vi "setSweep.vi"(8 "error in (no error)":errorcluster, 10 "Configure Sweep":T1 {"Channels"."Table" format="%#_1f"; "Channels"."Channel" min=1 max=128; "Channels"."Start" format="%#_6p"; "Channels"."End" format="%#_6p"; "Initial Wait (s)" format="%#_6p"}, 11 "Instrument.Lockin in":refnum<class "Instrument.Lockin.lvclass">) -> (0 "error out":errorcluster, 3 "Instrument.Lockin out":refnum<class "Instrument.Lockin.lvclass">)   [LabVIEW 2019, in "Instrument.Lockin.lvlib" / "Instrument.Lockin.lvclass"]
doc: "Configure Sweep mode"
uses:
  Instrument.Lockin.lvclass
  Instrument.DAQ/Typedefs/Sweep.Configuration--Cluster.ctl
  Instrument.DAQ/Typedefs/Sweep.Channel--Cluster--Array.ctl
  Instrument.DAQ/Typedefs/Sweep.Channel--Cluster.ctl
  Instrument.DAQ/Typedefs/Sweep.Pattern--Enum.ctl
  Typedefs/API/Lockin.Commands--Enum.ctl
  Instrument.DAQ/Instrument.DAQ.lvclass
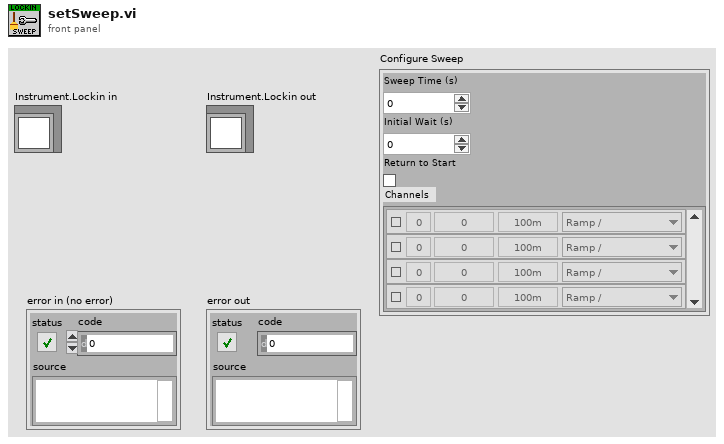
[diagram p1: front panel]
types:
  T1 = typedef "Instrument.Lockin.lvlib/Instrument.DAQ.lvclass/Sweep.Configuration--Cluster.ctl" = cluster{"Sweep Time (s)":dbl, "Initial Wait (s)":dbl, "Return to Start":bool, "Channels":T2}
  T2 = typedef "Instrument.Lockin.lvlib/Instrument.DAQ.lvclass/Sweep.Channel--Cluster--Array.ctl" = T3[]
  T3 = typedef "Instrument.Lockin.lvlib/Instrument.DAQ.lvclass/Sweep.Channel--Cluster.ctl" = cluster{"Enable?":bool, "Channel":u16, "Start":dbl, "End":dbl, "Pattern":T4, "Table":dbl[]}
  T4 = typedef "Instrument.Lockin.lvlib/Instrument.DAQ.lvclass/Sweep.Pattern--Enum.ctl" = enum16{"Ramp /", "Ramp /\\", "Smooth Ramp _/", "Smooth Ramp _/\\_", "Table"}
  T5 = typedef "Instrument.Lockin.lvlib/Instrument.Lockin.lvclass/Lockin.Commands--Enum.ctl" = enum16{"setAO", "setAO_Amplitude", "setAO_DC", "setAO_Frequency", "setAO_Phase", "setAO_Function", "setREF", "setREF_Frequency", "setREF_Phase", "setREF_TC", "setREF_Roll-Off", "setDAQ", "setSampling", "setState", "getState", "getAO", "getAI", "getResults", "getSampling", "getAOconfig", "getREFconfig", "setInputGain", "setOutputGain", "getInputGain", "getOutputGain", "setSamplingFsMode", "getSamplingFsMode", "setSweep", "setSweep_Time", "setSweep_Table", "getStatus", "getSweepResults", "getSweepWaveforms", "setLogMode"}
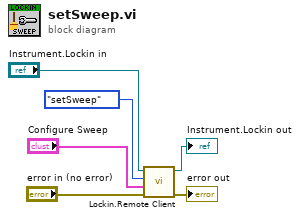
[diagram p0: block diagram]
diagram:
  n1 = call "Lockin.Remote Client.vi"("error in (no error)"="error in (no error)", "Data"="Configure Sweep", "Command"=Lockin.Commands--Enum."setSweep", "Instrument.Lockin in"="Instrument.Lockin in") -> ("error out"=→"error out":errorcluster, "Instrument.Lockin out"=→"Instrument.Lockin out":refnum<class "Instrument.Lockin.lvclass">)  [unwired: 5 in, 1 out]
